vi "(SubVI) Wang 97 Tether Calibration-using 7th order.vi"(6 "Set lower foce offset?":bool, 8 "stuckbead path (dialog if empty)":path, 9 "QPD signal":dbl[](array[numeric]), 10 "Stage Position":dbl[](array[numeric]), 11 "Fitting Cluster":T2={"cr (um)"=0.0, "yr (V)"=0.0, "trap height(nm)"=0.0, "bead radius(nm)"=520.0, "Length offset"=0.0, "Upper Force(pN)"=0.0, "cr shift (nm)"=0.0, "yr shift (mV)"=0.0, "LaserPower (mW)"=0.0, "conversion factor (V/um)"=0.0, "Stiffness (pN/nm)"=0.0154, "xDNA cut outside"=0.0, "Lower Force(pN)"=5.0, "c for zbd"=0.0}) -> (1 "Force":dbl[](array[numeric]), 2 "xDNA":dbl[](array[numeric]), 3 "output cluster":T2={"cr (um)"=0.0, "yr (V)"=0.0, "trap height(nm)"=0.0, "bead radius(nm)"=520.0, "Length offset"=0.0, "Upper Force(pN)"=0.0, "cr shift (nm)"=0.0, "yr shift (mV)"=0.0, "LaserPower (mW)"=0.0, "conversion factor (V/um)"=0.0, "Stiffness (pN/nm)"=0.0154, "xDNA cut outside"=0.0, "Lower Force(pN)"=5.0, "c for zbd"=0.0}, 4 "Xbead (nm)":dbl[](array[numeric]), 5 "zbd (nm)":dbl[](array[numeric]))   [LabVIEW 2014]
uses:
  WLC-Fitting Cluster.ctl
panel:
  out "XY Graph":T1(graph)
  out "Xst (nm)":dbl[](array[numeric])
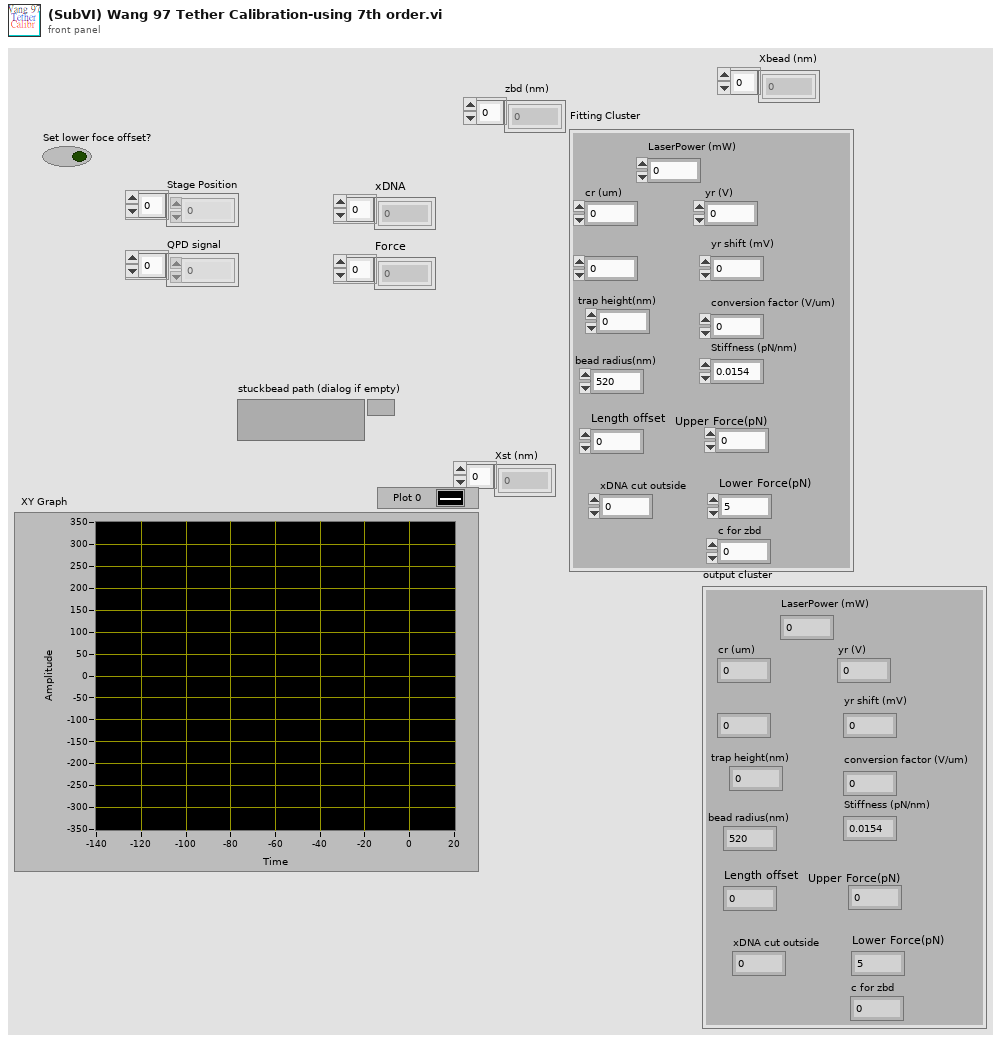
[diagram p1: front panel]
types:
  T1 = cluster{"Xbead (nm)":dbl[], "cut-full Force":dbl[]}
  T2 = typedef "WLC-Fitting Cluster.ctl" = cluster{"cr (um)":dbl, "yr (V)":dbl, "trap height(nm)":dbl, "bead radius(nm)":dbl, "Length offset":dbl, "Upper Force(pN)":dbl, "cr shift (nm)":dbl, "yr shift (mV)":dbl, "LaserPower (mW)":dbl, "conversion factor (V/um)":dbl, "Stiffness (pN/nm)":dbl, "xDNA cut outside":dbl, "Lower Force(pN)":dbl, "c for zbd":dbl}
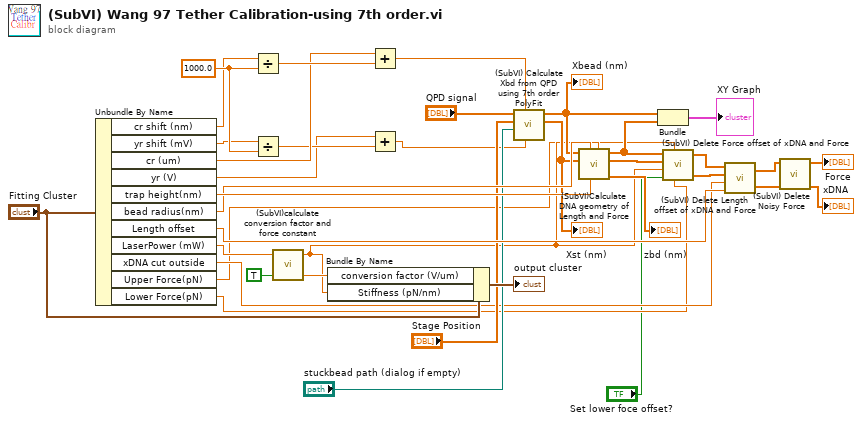
[diagram p0: block diagram]
diagram:
  w31 = 1000.0 ("y")
  n1 = Unbundle By Name("Fitting Cluster") -> ("cr shift (nm)"=w30:dbl, "yr shift (mV)"=w29:dbl, "cr (um)"=w27:dbl, "yr (V)"=w25:dbl, "trap height(nm)"=w34:dbl, "bead radius(nm)"=w33:dbl, "Length offset"=w32:dbl, "LaserPower (mW)"=w24:dbl, "xDNA cut outside"=w4:dbl, "Upper Force(pN)"=w3:dbl, "Lower Force(pN)"=w2:dbl)
  n2 = Divide(x=w30, y=w31) -> (x/y=w28:dbl)
  n3 = Divide(x=w29, y=w31) -> (x/y=w26:dbl)
  n4 = call "(SubVI)calculate conversion factor and force constant.vi"("X=T\nY=F"=TRUE ("X=T\nY=F"), "laser power (mW)"=w24) -> ("conversion factor (V/um)"=w22:dbl, "force constant (pN/nm)"=w10:dbl)  [unwired: 2 in]
  n5 = Bundle By Name(cluster="Fitting Cluster", "conversion factor (V/um)"=w22, "Stiffness (pN/nm)"=w10) -> (→"output cluster":T2)
  n6 = Add(x=w27, y=w28) -> (x+y=w16:dbl)
  n7 = Add(x=w25, y=w26) -> (x+y=w15:dbl)
  n8 = call "(SubVI) Calculate Xbd from QPD using 7th order PolyFit.vi"("yr (V)"=w15, "cr (um)"=w16, "file path (dialog if empty)"="stuckbead path (dialog if empty)", "Stage Position (um)"="Stage Position", "QPD Signal (V)"="QPD signal") -> ("Xst (nm)"=w18:dbl[], "Xbead (nm)"=w12:dbl[])  [unwired: 3 in]
  "Xst (nm)" <- w18
  "Xbead (nm)" <- w12
  n9 = call "(SubVI)Calculate DNA geometry of Length and Force.vi"("Force constant (pN/nm)"=w10, "trap height(nm)"=w34, "bead radius(nm)"=w33, "Xst"=w18, "Xbd"=w12) -> ("zbd (nm)"=→"zbd (nm)":dbl[], "xDNA"=w37:dbl[], "Force"=w11:dbl[])  [unwired: 4 in]
  n10 = Bundle("Xbead (nm)"=w12, "Force"=w11) -> (→"XY Graph":cluster{"Xbead (nm)":dbl[], "Force":dbl[]})  [unwired: 1 in]
  n11 = call "(SubVI) Delete Force offset of xDNA and Force.vi"("Force"=w11, "Upper Force (pN)"=w3, "xDNA"=w37, "force constant"=w10, "Lower Force (pN)"=w2, "Set lower foce offset?"="Set lower foce offset?") -> ("cut-full Force"=w36:dbl[], "cut-full xDNA"=w35:dbl[])  [unwired: 1 in]
  n12 = call "(SubVI) Delete Length offset of xDNA and Force.vi"("Length offset"=w32, "xDNA cut outside (nm)"=w4, "xDNA"=w35, "Force"=w36) -> ("cut-full xDNA"=w7:dbl[], "cut-full Force"=w8:dbl[])
  n13 = call "(SubVI) Delete Noisy Force.vi"("xDNA"=w7, "Force"=w8) -> ("xDNA-cut"=→"xDNA":dbl[], "Force-cut"=→"Force":dbl[])  [unwired: 4 in]
